vi "Labview_USB_I2C_SlaveWriteRead.vi"() -> ()   [LabVIEW 2010]
uses:
  Labview_USB_I2C_AM2321B/lib/labview_32bit/ControlI2C/Ginkgo_Driver.dll
panel:
  out "Flag(T:read;F:write)":bool=TRUE
  in  "Constant":T1={"DevType"=1, "DevIndex"=0, "I2CIndex"=0}
  in  "pInitConfig":T2={"MasterMode"=1, "ControlMode"=1, "AddrType"=7, "SubAddrWidth"=0, "Addr"=0, "@dummy control@"=0, "@dummy control@"=0, "ClockSpeed"=0}
  out "error out":errorcluster
  in  "Read":bool
  in  "Write":bool
  in  "Slave Addr(Hex)":u8 format="%x"
  out "Read Data(Hex)":string
  in  "Channel Index":u16(ring) items=["0", "1"]
  in  "Write Data(Hex)":string
  in  "Device Index":u16(ring) items=["0", "1", "2", "3", "4", "5", "6", "7", "8", "9"]
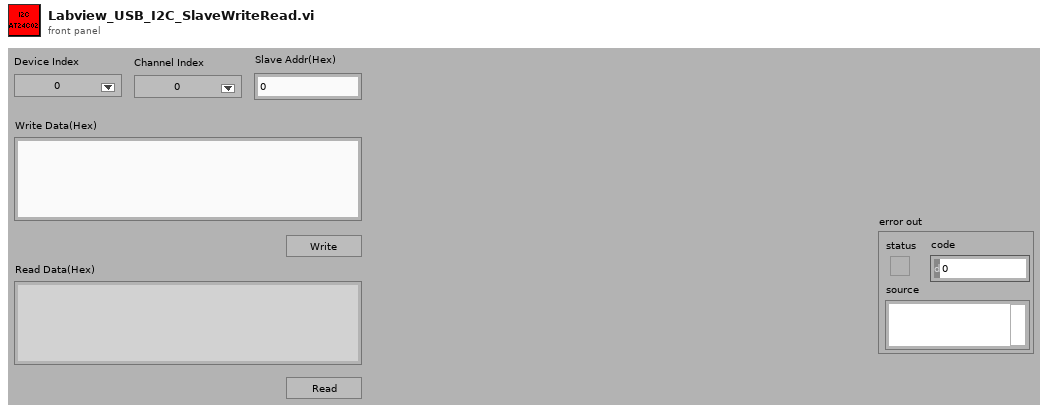
[diagram p1: front panel]
types:
  T1 = cluster{"DevType":i32, "DevIndex":i32, "I2CIndex":i32}
  T2 = cluster{"MasterMode":u8, "ControlMode":u8, "AddrType":u8, "SubAddrWidth":u8, "Addr":u16, "@dummy control@":i8, "@dummy control@":i8, "ClockSpeed":u32}
  T3 = enum16{"Init", "Write", "Read", "Idel", "Close", "Error"}
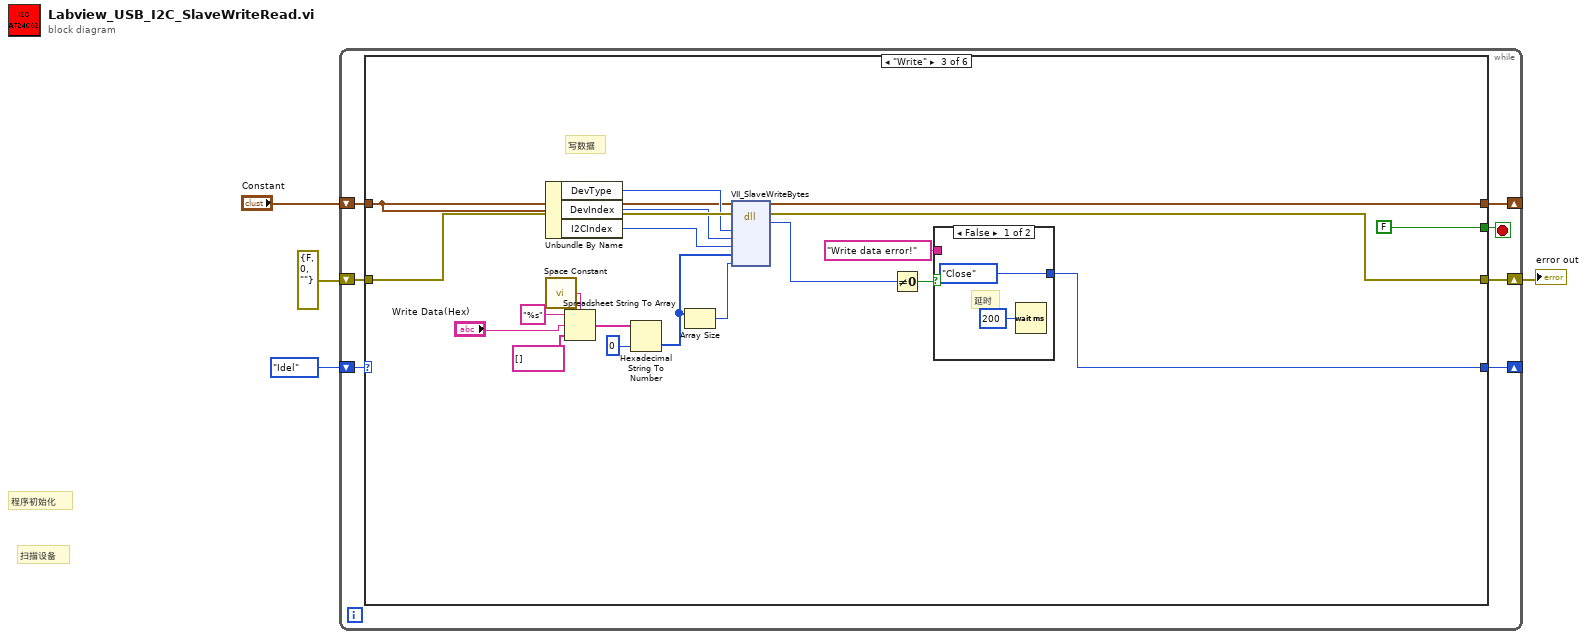
[diagram p0: block diagram]
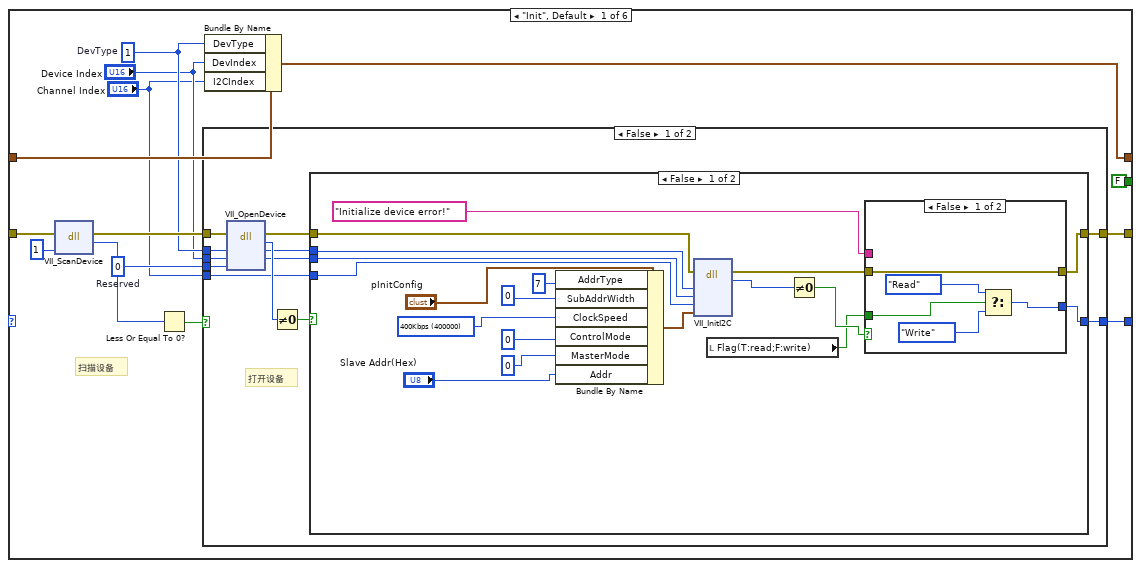
[diagram p2: hidden frame]
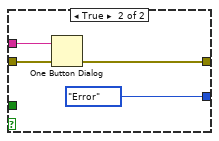
[diagram p3: hidden frame]
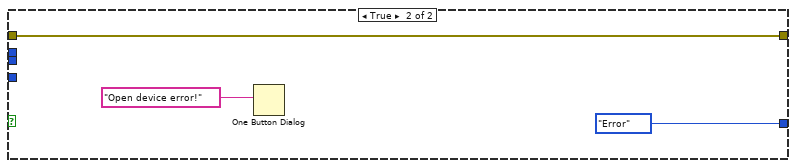
[diagram p4: hidden frame]
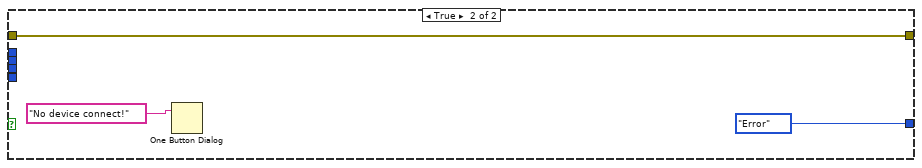
[diagram p5: hidden frame]
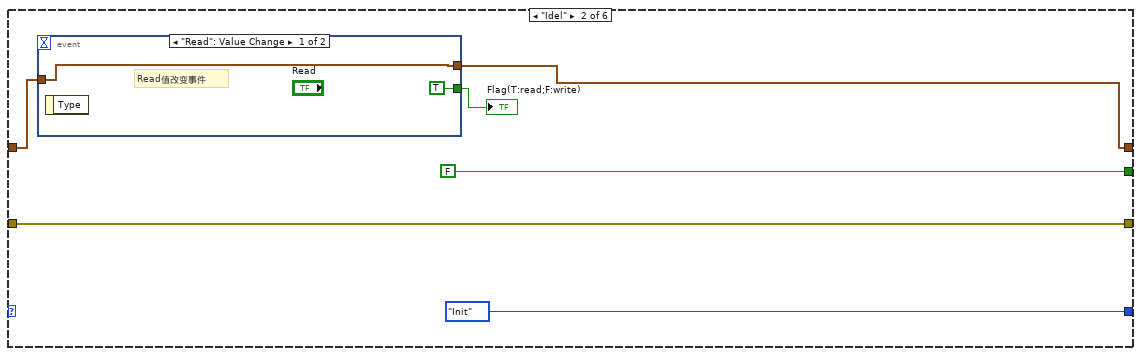
[diagram p6: hidden frame]
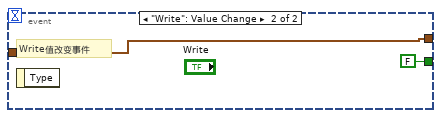
[diagram p7: hidden frame]
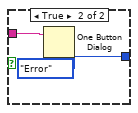
[diagram p8: hidden frame]
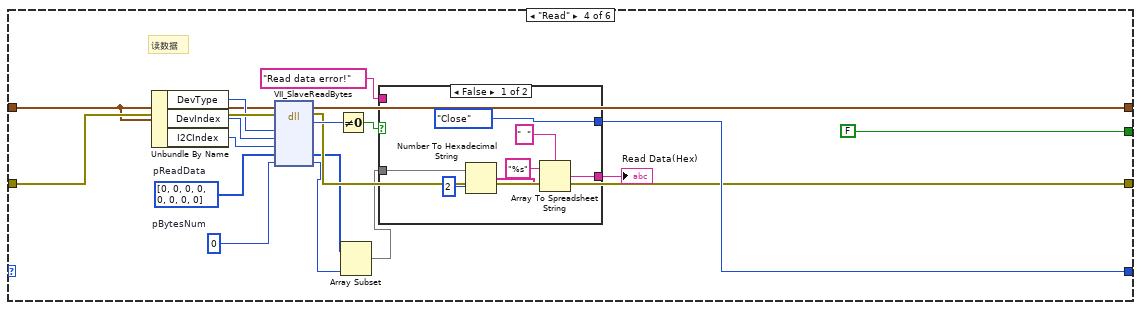
[diagram p9: hidden frame]
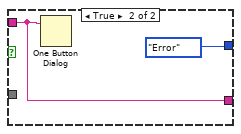
[diagram p10: hidden frame]
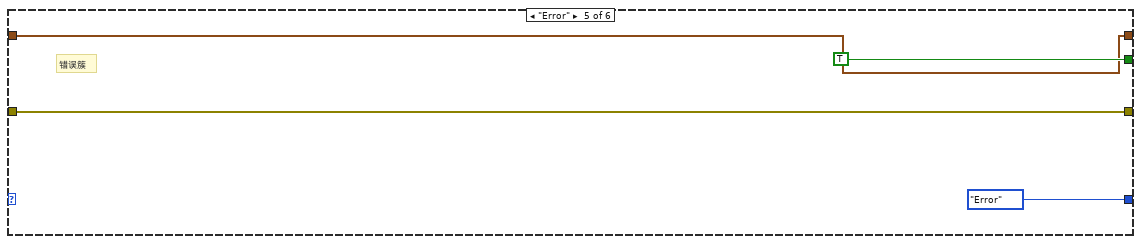
[diagram p11: hidden frame]
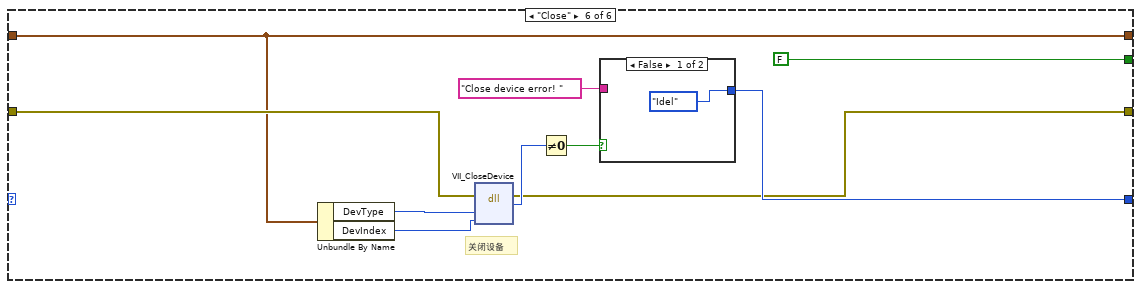
[diagram p12: hidden frame]
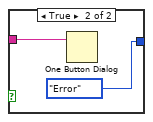
[diagram p13: hidden frame]
diagram:
  # "扫描设备"
  # "程序初始化"
  n1 = while {
    shift-right: [w11] -> _
    shift-left: T3."Idel" ("Enum") -> [w10]
    shift-right: [w8] -> w2
    shift-left: errorcluster {"status"=FALSE, "code"=0, "source"=""} ("error out") -> [w7]
    shift-right: [w5] -> _
    shift-left: "Constant" -> [w6]
    stop <- w9 stop-if-true
    n2 = case shown="\"Write\"" w10 {
      tunnel: [w17 T3."Init" ("Enum") w91 w113 T3."Error" ("Enum") w139] -> w11
      tunnel: [FALSE ("stop") FALSE ("stop") FALSE ("stop") FALSE ("stop") TRUE ("stop") FALSE ("stop")] -> w9
      tunnel: [w18 w75 w90 w112 w132 w138] -> w8
      tunnel: w7 -> [w19 w75 w98 w119 w132 w137]
      tunnel: w6 -> [w16 w74 w94 w111 w130 w136]
      tunnel: [w12 w73 w94 w111 w130 w136] -> w5
      frame "Init", Default {
        w20 = 0  # Reserved
        w15 = 1  # DevType
        # "扫描设备"
        n3 = dll-call lib="E:/Project/vt_ginkgo_examples/trunk/Labview/Ginkgo I2C/Labview_USB_I2C_AM2321B/lib/labview_32bit/ControlI2C/Ginkgo_Driver.dll" fn="VII_ScanDevice"(error in=w19, "NeedInit"=u8 1) -> (error out=w21:errorcluster, "return type"=w23:i32)  [unwired: 3 in, 1 out]
        n4 = Less Or Equal To 0?(x=w23) -> (x <= 0?=w22:bool)
        n5 = case shown="False" w22 {
          tunnel: [w31 T3."Error" ("Enum")] -> w17
          tunnel: w21 -> [w35 w69]
          tunnel: w20 -> [w34 _]
          tunnel: "Device Index" -> [w33 _]
          tunnel: w15 -> [w32 _]
          tunnel: [w27 w69] -> w18
          tunnel: "Channel Index" -> [w26 _]
          frame False {
            # "打开设备"
            n6 = dll-call lib="E:/Project/vt_ginkgo_examples/trunk/Labview/Ginkgo I2C/Labview_USB_I2C_AM2321B/lib/labview_32bit/ControlI2C/Ginkgo_Driver.dll" fn="VII_OpenDevice"(error in=w35, "DevType"=w32, "DevIndex"=w33, "Reserved"=w34) -> (error out=w30:errorcluster, "return type"=w36:i32, "DevType"=w29:i32, "DevIndex"=w28:i32)  [unwired: 3 in, 1 out]
            n7 = Not Equal To 0?(x=w36) -> (x != 0?=w37:bool)
            n8 = case shown="False" w37 {
              tunnel: [w45 T3."Error" ("Enum")] -> w31
              tunnel: w30 -> [w48 w66]
              tunnel: w29 -> [w47 _]
              tunnel: w28 -> [w46 _]
              tunnel: [w44 w66] -> w27
              tunnel: w26 -> [w43 _]
              frame False {
                w52 = u32 400000 items=["800Kbps"=800000, "400Kbps"=400000, "200Kbps"=200000, "100Kbps"=100000, "50Kbps"=50000] ("Speed")
                n9 = Bundle By Name(cluster="pInitConfig", "AddrType"=u8 7, "SubAddrWidth"=u8 0, "ClockSpeed"=w52, "ControlMode"=u8 0, "MasterMode"=u8 0, "Addr"="Slave Addr(Hex)") -> (w54:T2)
                n10 = dll-call lib="E:/Project/vt_ginkgo_examples/trunk/Labview/Ginkgo I2C/Labview_USB_I2C_AM2321B/lib/labview_32bit/ControlI2C/Ginkgo_Driver.dll" fn="VII_InitI2C"(error in=w48, "DevType"=w47, "DevIndex"=w46, "I2CIndex"=w43, "pInitConfig"=w54) -> (error out=w51:errorcluster, "return type"=w56:i32)  [unwired: 6 in, 1 out]
                n11 = local read "Flag(T:read;F:write)"() -> (w39:bool)
                n12 = Not Equal To 0?(x=w56) -> (x != 0?=w55:bool)
                n13 = case shown="False" w55 {
                  tunnel: "Initialize device error!" ("message") -> [_ w64]
                  tunnel: [w57 T3."Error" ("Enum")] -> w45
                  tunnel: w51 -> [w61 w62]
                  tunnel: [w61 w62] -> w44
                  tunnel: w39 -> [w60 _]
                  frame False {
                    n14 = Select(t=T3."Read" ("Enum"), s=w60, f=T3."Write" ("Enum")) -> (s? t:f=w57:T3)
                  }
                  frame True {
                    n15 = One Button Dialog(message=w64) -> ()  [unwired: 1 in, 1 out]
                  }
                }
              }
              frame True {
                n16 = One Button Dialog(message="Open device error!") -> ()  [unwired: 1 in, 1 out]
              }
            }
          }
          frame True {
            n17 = One Button Dialog(message="No device connect!") -> ()  [unwired: 1 in, 1 out]
          }
        }
        n18 = Bundle By Name(cluster=w16, "DevType"=w15, "DevIndex"="Device Index", "I2CIndex"="Channel Index") -> (w12:T1)
      }
      frame "Idel" {
        n19 = event shown="[0] \"Read\": Value Change" {
          selector: _ -> [_ _]
          dyn-events: _ -> [_ _]
          timeout: _ -> [_ _]
          tunnel: w74 -> [w78 w80]
          tunnel: [w78 w80] -> w73
          tunnel: [TRUE ("Read") FALSE ("Read")] -> w71
          event "Read": Value Change {
            # "Read值改变事件"
            n20 = event-data() -> ()  [unwired: 1 in, 1 out]
          }
          event "Write": Value Change {
            # "Write值改变事件"
            n21 = event-data() -> ()  [unwired: 1 in, 1 out]
          }
        }
        "Flag(T:read;F:write)" <- w71
      }
      frame "Write" {
        # "写数据"
        n22 = Unbundle By Name(w94) -> ("DevType"=w97:i32, "DevIndex"=w96:i32, "I2CIndex"=w95:i32)
        n23 = call <vilib>:"Space Constant.vi"() -> ("String"=w83:string)
        n24 = Spreadsheet String To Array(delimiter (Tab)=w83, format string="%s", spreadsheet string="Write Data(Hex)", array type (2D Dbl)=string[] []) -> (array=w86:string[])
        n25 = Hexadecimal String To Number(string=w86, default (0uL)=u8 0 ("default (0 U32)")) -> (number=w81:u8[])  [unwired: 1 in, 1 out]
        n26 = Array Size(array=w81) -> (size(s)=w88:i32)
        n27 = dll-call lib="E:/Project/vt_ginkgo_examples/trunk/Labview/Ginkgo I2C/Labview_USB_I2C_AM2321B/lib/labview_32bit/ControlI2C/Ginkgo_Driver.dll" fn="VII_SlaveWriteBytes"(error in=w98, "DevType"=w97, "DevIndex"=w96, "I2CIndex"=w95, "pWriteData"=w81, "Len"=w88) -> (error out=w90:errorcluster, "return type"=w92:i32)  [unwired: 7 in, 1 out]
        n28 = Not Equal To 0?(x=w92) -> (x != 0?=w89:bool)
        n29 = case shown="False" w89 {
          tunnel: "Write data error!" ("message") -> [_ w103]
          tunnel: [T3."Close" ("Enum") T3."Error" ("Enum")] -> w91
          frame False {
            # "延时"
            n30 = Wait (ms)(milliseconds to wait=u32 200) -> ()  [unwired: 1 out]
          }
          frame True {
            n31 = One Button Dialog(message=w103) -> ()  [unwired: 1 in, 1 out]
          }
        }
      }
      frame "Read" {
        w105 = 0  # pBytesNum
        w108 = u8[] [0, 0, 0, 0, 0, 0, 0, 0]  # pReadData
        # "读数据"
        n32 = Unbundle By Name(w111) -> ("DevType"=w118:i32, "DevIndex"=w117:i32, "I2CIndex"=w116:i32)
        n33 = dll-call lib="E:/Project/vt_ginkgo_examples/trunk/Labview/Ginkgo I2C/Labview_USB_I2C_AM2321B/lib/labview_32bit/ControlI2C/Ginkgo_Driver.dll" fn="VII_SlaveReadBytes"(error in=w119, "DevType"=w118, "DevIndex"=w117, "I2CIndex"=w116, "pReadData"=w108, "pLen"=w105) -> (error out=w112:errorcluster, "return type"=w115:i32, "pReadData"=w107:u8[], "pLen"=w104:u16)  [unwired: 5 in, 1 out]
        n34 = Not Equal To 0?(x=w115) -> (x != 0?=w110:bool)
        n35 = Array Subset(array=w107, length=w104) -> (w106:u8[])  [unwired: 1 in]
        n36 = case shown="False" w110 {
          tunnel: "Read data error!" ("message") -> [_ w128]
          tunnel: [T3."Close" ("Enum") T3."Error" ("Enum")] -> w113
          tunnel: w106 -> [w122 _]
          tunnel: [w121 w128] -> w109
          frame False {
            n37 = Number To Hexadecimal String(1:i16 2 ("width (-)"), 2:w122) -> (0:w124:string[])
            n38 = Array To Spreadsheet String(delimiter (Tab)="  ", array=w124, 3:"%s" ("format string")) -> (spreadsheet string=w121:string)
          }
          frame True {
            n39 = One Button Dialog(message=w128) -> ()  [unwired: 1 in, 1 out]
          }
        }
        "Read Data(Hex)" <- w109
      }
      frame "Error" {
        # "错误簇"
      }
      frame "Close" {
        # "关闭设备"
        n40 = Unbundle By Name(w136) -> ("DevType"=w135:i32, "DevIndex"=w134:i32)
        n41 = dll-call lib="E:/Project/vt_ginkgo_examples/trunk/Labview/Ginkgo I2C/Labview_USB_I2C_AM2321B/lib/labview_32bit/ControlI2C/Ginkgo_Driver.dll" fn="VII_CloseDevice"(error in=w137, "DevType"=w135, "DevIndex"=w134) -> (error out=w138:errorcluster, "return type"=w141:i32)  [unwired: 4 in, 1 out]
        n42 = Not Equal To 0?(x=w141) -> (x != 0?=w140:bool)
        n43 = case shown="False" w140 {
          tunnel: "Close device error! " ("message") -> [_ w146]
          tunnel: [T3."Idel" ("Enum") T3."Error" ("Enum")] -> w139
          frame False {
          }
          frame True {
            n44 = One Button Dialog(message=w146) -> ()  [unwired: 1 in, 1 out]
          }
        }
      }
    }
  }
  "error out" <- w2
